vi "QE Reset.vi"(8 "Error In":errorcluster, 10 "QE Channels":u8[](array[numeric]), 11 "LINX Device Config":T1) -> (0 "Error Out":errorcluster, 3 "LINX Device Config":T1)   [LabVIEW 2013, in "LVH-LINX.lvlib" / "Device.lvlib"]
uses:
  Device.lvlib
  Type Defs/LINX Device Config.ctl
  Type Defs/Interface.ctl
  Type Defs/TCP Config.ctl
  Type Defs/Channels.ctl
  Type Defs/Error Type.ctl
  LVH-LINX.lvlib
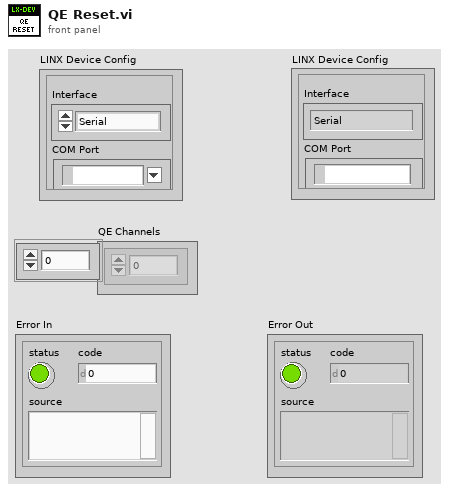
[diagram p1: front panel]
types:
  T1 = typedef "LVH-LINX.lvlib/Device.lvlib/LINX Device Config.ctl" = cluster{"Interface":T2, "COM Port":refnum<visa-resource-name>, "TCP Configuration":T3, "Device Family":u8, "Device ID":u8, "Device Name":string, "TCP Ref":refnum<k5>, "Channels":T4}
  T2 = typedef "LVH-LINX.lvlib/Interface.ctl" = enum16{"Serial", "TCP"}
  T3 = typedef "LVH-LINX.lvlib/Device.lvlib/TCP Config.ctl" = cluster{"IP Address":string, "Port":u16}
  T4 = typedef "LVH-LINX.lvlib/Channels.ctl" = cluster{"DI Channels":u8[], "DO Channels":u8[], "AI":u8[], "AO":u8[], "PWM":u8[], "QE":u8[], "UART":u8[], "I2C 2":u8[], "SPI":u8[], "CAN":u8[], "AI Ref (V)":dbl, "AO Resolution (Bits)":u8, "AO Ref (V)":dbl}
  T5 = typedef "LVH-LINX.lvlib/Error Type.ctl" = enum16{"Unknown", "Timeout", "Corrupt Return Packet", "Unable To Connect", "Command Not Supported", "Channel DNE", "Invalid COM Config", "Firmware Version Mismatch", "myRIO Support"}
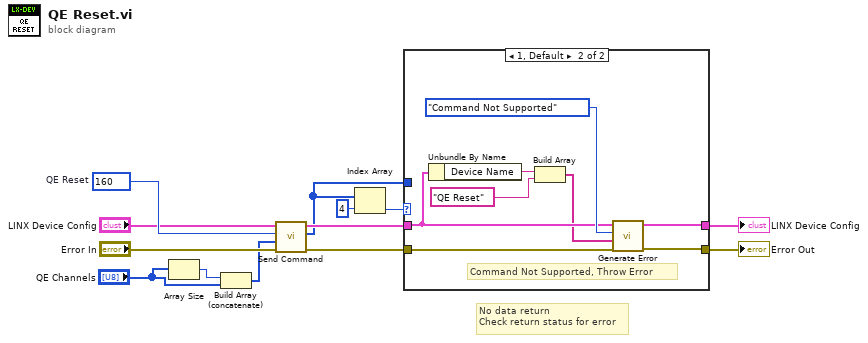
[diagram p0: block diagram]
diagram:
  w12 = u16 160  # QE Reset
  # "No data return\nCheck return status for error"
  n1 = Array Size(array="QE Channels") -> (size(s)=w3:i32)
  n2 = Build Array (concatenate)(w3, "QE Channels") -> (w2:i32[])
  n3 = call "Send Command.vi"("Error In"="Error In", "ARGS"=w2, "CMD"=w12, "LINX Device Config"="LINX Device Config") -> ("Error Out"=w5:errorcluster, "Response"=w4:u8[], "LINX Device Config"=w7:T1)  [unwired: 4 in, 1 out]
  n4 = Index Array(array=w4, index=4) -> (element=w9:u8)
  n5 = case shown="1, Default" w9 {
    tunnel: [w15 w21] -> w8
    tunnel: w7 -> [w15 w17]
    tunnel: [w14 w22] -> w6
    tunnel: w5 -> [w14 w23]
    tunnel: w4 -> [_ _]
    frame 0 {
      # "Status OK, Process Data"
    }
    frame 1, Default {
      # "Command Not Supported, Throw Error"
      n6 = Unbundle By Name(w17) -> ("Device Name"=w19:string)
      n7 = Build Array(w19, "QE Reset") -> (w16:string[])
      n8 = call "Generate Error.vi"("Error In"=w23, "Arguments"=w16, "Error Type"=Error_Type."Command Not Supported", "LINX Device Config"=w17) -> ("Error Out"=w22:errorcluster, "LINX Device Config"=w21:T1)  [unwired: 6 in]
    }
  }
  "Error Out" <- w6
  "LINX Device Config" <- w8
